vi "Scripting Save object.vi"(7 "Object type":T1=21751 items=[".NET Container"=2125, ".NET Refnum"=3441, "2D Picture"=3508, "3D Picture"=23776, "ActiveX Container"=2072, "Application Refnum"=3412, "Array (classic)"=3300, "Array (modern)"=21608, "Array Interface Control"=23777, "Atmospheric Tank (classic)"=3070, "Atmospheric Tank (modern)"=21751, "Automation Refnum"=3410, "Bin 1"=3073, "Bin 2"=21755, "Byte Stream File Refnum"=3408, "CAN Channel (classic)"=3340, "CAN Channel (modern)"=21817, "CAN Channel (system)"=21966, "CAN Interface (classic)"=3339, "CAN Interface (modern)"=21815, "CAN Interface (system)"=21964, "CAN Task (classic)"=3470, "CAN Task (modern)"=21789, "CAN Task (system)"=21963, "Cancel Button (modern)"=21739, "Cancel Button (system)"=3131, "Checkbox (classic)"=3117, "CheckBox (modern)"=21924, "Checkbox (system)"=3132, "Cluster (classic)"=3400, "Cluster (modern)"=21607, "Color Box"=3013, "Color Box Thin Border"=2905, "Color Ramp"=3022, "Combo Box (classic)"=3304, "Combo Box (modern)"=21604, "Combo Box (system)"=21917, "Control Refnum"=3419, "DAQmx Analog Trigger Source (classic)"=3336, "DAQmx Analog Trigger Source (modern)"=21774, "DAQmx Analog Trigger Source (system)"=21951, "DAQmx Device Name (classic)"=3318, "DAQmx Device Name (modern)"=21773, "DAQmx Device Name (system)"=21950, "DAQmx Global Channel (classic)"=3443, "DAQmx Global Channel (modern)"=21770, "DAQmx Global Channel (system)"=21957, "DAQmx Physical Channel (classic)"=3335, "DAQmx Physical Channel (modern)"=21777, "DAQmx Physical Channel (system)"=21954, "DAQmx Scale Name (classic)"=3317, "DAQmx Scale Name (modern)"=21775, "DAQmx Scale Name (system)"=21952, "DAQmx Switch (classic)"=3337, "DAQmx Switch (modern)"=21776, "DAQmx Switch (system)"=21953, "DAQmx Task Name (classic)"=3442, "DAQmx Task Name (modern)"=21778, "DAQmx Task Name (system)"=21959, "DAQmx Terminal (classic)"=3319, "DAQmx Terminal (modern)"=21781, "DAQmx Terminal (system)"=21955, "Data Log File Refnum"=3402, "DataSocket Refnum"=3417, "Device Refnum"=3405, "Dial (classic)"=3050, "Dial (modern)"=21732, "Digital Data (classic)"=3210, "Digital Data (modern)"=21216, "Digital Waveform Graph (classic)"=3511, "Digital Waveform Graph (modern)"=21718, "Dlg Horiz Scrollbar"=21905, "Dlg Numeric 1"=2100, "Dlg Numeric 2"=3006, "Dlg String"=2110, "Dlg Vert Scrollbar"=21906, "Down Arrow"=3824, "Down Bow Valve (flat)"=3707, "Down Bow Valve (outline)"=3807, "Down Bow Valve (shaded)"=21767, "Down Rect Valve (flat)"=3706, "Down Rect Valve (outline)"=3806, "Down Rect Valve (shaded)"=21766, "Down Tee (flat)"=3818, "Down Tee (shaded)"=3718, "Enum (classic)"=3023, "Enum (modern)"=21605, "Enum (system)"=3062, "Event Callback Refnum"=3435, "Exchanger"=3828, "FieldPoint IO Point (classic)"=3439, "FieldPoint IO Point (modern)"=21784, "FIFO Refnum"=3474, "File Path Control (classic)"=3203, "File Path Control (modern)"=21730, "File Path Control (system)"=21922, "File Path Indicator (classic)"=3204, "File Path Indicator (modern)"=21731, "Flat Box"=3602, "Flat Circle"=3605, "Flat Down Triangle"=3623, "Flat Frame"=3608, "Flat Left Triangle"=3620, "Flat Right Triangle"=3621, "Flat Round Button"=3102, "Flat Rounded Box"=3611, "Flat Sequence Structure"=2069, "Flat Square Button"=3103, "Flat Up Triangle"=3622, "Framed Color Box (classic)"=3008, "Framed Color Box (modern)"=21019, "Furnace"=3829, "Gauge (classic)"=3040, "Gauge (modern)"=21009, "Hopper 1"=21754, "Hopper 2"=3072, "Horiz Line"=3821, "Horiz Pipe (flat)"=3810, "Horiz Pipe (shaded)"=3710, "Horizontal Button Box"=3636, "Horizontal Fill Slide (classic)"=3012, "Horizontal Fill Slide (modern)"=21100, "Horizontal Graduated Bar"=21106, "Horizontal Pointer Slide (classic)"=3011, "Horizontal Pointer Slide (modern)"=21101, "Horizontal Pointer Slide (system)"=21902, "Horizontal Progress Bar (modern)"=21102, "Horizontal Progress Bar (system)"=21910, "Horizontal Scrollbar"=21110, "Horizontal Slide (classic)"=3010, "Horizontal Slide (system)"=21904, "Horizontal Slide Switch"=3114, "Horizontal Smooth Box"=3633, "Horizontal Splitter Bar (Classic)"=21863, "Horizontal Splitter Bar (System)"=21865, "Horizontal Switch"=3108, "Horizontal Tank"=3071, "Horizontal Toggle Switch (classic)"=3110, "Horizontal Toggle Switch (modern)"=21700, "IMAQ Session"=3415, "Intensity Chart (classic)"=3509, "Intensity Chart (modern)"=21719, "Intensity Graph (classic)"=3510, "Intensity Graph (modern)"=21720, "IrDA Network Connection Refnum"=3450, "IVI Logical Name (classic)"=3414, "IVI Logical Name (modern)"=21736, "Knob (classic)"=3005, "Knob (modern)"=21000, "Label (modern)"=21960, "Label (system)"=21961, "Labeled Oblong Button"=3125, "Labeled Rectangular Button"=3124, "Labeled Round Button"=3122, "Labeled Square Button"=3123, "LED Button"=3116, "Left Arrow"=3826, "Left Bow Valve (flat)"=3701, "Left Bow Valve (outline)"=3801, "Left Bow Valve (shaded)"=21761, "Left Down Elbow (flat)"=3811, "Left Down Elbow (shaded)"=3711, "Left Pump (flat)"=3813, "Left Pump (shaded)"=3713, "Left Rect Valve (flat)"=3700, "Left Rect Valve (outline)"=3800, "Left Rect Valve (shaded)"=21760, "Left Tee (flat)"=3809, "Left Tee (shaded)"=3709, "Left Up Elbow (flat)"=3808, "Left Up Elbow (shaded)"=3708, "Line (chiseled, system)"=3632, "Line (chiseled, thick)"=3630, "Line (chiseled, thin)"=3627, "Line (thick)"=3629, "Line (thin)"=3626, "Line with Arrow (thick)"=3631, "Line with Arrow (thin)"=3628, "Listbox (classic)"=21806, "Listbox (modern)"=21792, "Listbox (system)"=21805, "Lowered Box (thick)"=3635, "Lowered Rounded Box"=3638, "Menu Refnum"=3413, "Menu Ring (classic)"=3018, "Menu Ring (modern)"=21600, "Menu-Popup Ring"=3017, "Meter (classic)"=3030, "Meter (modern)"=21008, "Mixed Checkbox (system)"=21333, "Mixed Signal Graph"=21721, "Motion Resource (classic)"=3448, "Motion Resource (modern)"=21787, "Motor (flat)"=3820, "Motor (shaded)"=3720, "Multi-Segment Pipe"=23780, "Multicolumn Listbox (classic)"=21799, "Multicolumn Listbox (modern)"=21791, "Multicolumn Listbox (system)"=21798, "Notifier Refnum"=3423, "Numeric Control (classic)"=3000, "Numeric Control (modern)"=21003, "Numeric Control (system)"=21919, "Numeric Indicator (classic)"=3001, "Numeric Indicator (modern)"=21004, "Occurrence Refnum"=3406, "OK Button (modern)"=21738, "OK Button (system)"=3130, "Open Application Reference"=8012, "Open VI Object Reference"=8013, "Open VI Reference"=8010, "PassControl"=1968, "Pict Ring (classic)"=3015, "Pict Ring (modern)"=21602, "Pict Ring (system)"=21925, "PixMap"=3505, "PixMap (warning: dangerous)"=3507, "Platform Flat Square Button"=3134, "Plug-In Control"=21820, "Preserve Run-Time Class"=8018, "Pressure Tank (flat)"=3075, "Pressure Tank (shaded)"=21753, "Preview Queue Element"=9112, "Pulldown Menu Ring"=3061, "Push Button"=21001, "Queue Refnum"=3424, "Radio Button (system)"=3133, "Radio Buttons (classic)"=22003, "Radio Buttons (modern)"=22001, "Radio Buttons (system)"=22002, "Raised Box (classic)"=3600, "Raised Box (modern)"=3637, "Raised Circle"=3603, "Raised Down Triangle"=3615, "Raised Frame"=3606, "Raised Left Triangle"=3612, "Raised Right Triangle"=3613, "Raised Rounded Box"=3609, "Raised Up Triangle"=3614, "Recessed Box"=3601, "Recessed Circle"=3604, "Recessed Down Triangle"=3619, "Recessed Frame (modern)"=3607, "Recessed Frame (system)"=3624, "Recessed Left Triangle"=3616, "Recessed Menu Ring"=3019, "Recessed Right Triangle"=3617, "Recessed Rounded Box"=3610, "Recessed Up Triangle"=3618, "RecomposeUnlockDataValRef (warning: dangerous)"=2407, "Rectangular Stop Button"=3128, "Right Arrow"=3825, "Right Bow Valve (flat)"=3705, "Right Bow Valve (outline)"=3805, "Right Bow Valve (shaded)"=21765, "Right Down Elbow (flat)"=3817, "Right Down Elbow (shaded)"=3717, "Right Pump (flat)"=3819, "Right Pump (shaded)"=3719, "Right Rect Valve (flat)"=3704, "Right Rect Valve (outline)"=3804, "Right Rect Valve (shaded)"=21764, "Right Tee (flat)"=3815, "Right Tee (shaded)"=3715, "Right Up Elbow (flat)"=3814, "Right Up Elbow (shaded)"=3714, "Rocker"=21002, "Rotary Feeder"=3830, "Round Button"=3100, "Round LED (classic)"=3120, "Round LED (modern)"=21012, "Round Light"=3104, "Round Push Button"=3118, "Round Push Button (profile)"=3112, "Round Radio Button"=3106, "Round Stop Button"=3127, "Shared Variable Control (classic)"=3472, "Shared Variable Control (modern)"=21814, "Simple Horizontal Slide"=3003, "Simple Numeric"=2900, "Simple String"=2115, "Simple Vertical Slide"=3002, "Slide Switch"=21011, "Spin Control (system)"=21900, "Split Button"=21020, "Split Number"=1170, "Square Button"=3101, "Square LED (classic)"=3121, "Square LED (modern)"=21013, "Square Light"=3105, "Square Push Button"=3119, "Square Push Button (profile)"=3113, "Square Radio Button"=3107, "Static VI Reference"=2084, "Stop"=1350, "Stop Button"=21230, "Stop Stream"=23807, "String Control (classic)"=3200, "String Control (modern)"=21701, "String Control (system)"=21920, "String Indicator (classic)"=3201, "String Indicator (modern)"=21702, "SubPanel (Classic)"=21811, "SubPanel (System)"=21823, "Tab Control (classic)"=3330, "Tab Control (modern)"=3332, "Tab Control (system)"=3331, "Table (classic)"=21796, "Table (modern)"=21790, "Table (system)"=21797, "Tag Attribute Ring"=2063, "Tank (classic)"=3020, "Tank (modern)"=21006, "TCP Network Connection Refnum"=3407, "Text & Pict Ring (classic)"=3016, "Text & Pict Ring (modern)"=21603, "Text Button"=21015, "Text Ring (classic)"=3014, "Text Ring (modern)"=21601, "Text Ring (system)"=3060, "Thermometer (classic)"=3021, "Thermometer (modern)"=21007, "Time Stamp Control (classic)"=5555, "Time Stamp Control (modern)"=21913, "Time Stamp Control (system)"=21967, "Time Stamp Indicator (classic)"=5556, "Time Stamp Indicator (modern)"=21914, "Tree (classic)"=21819, "Tree (modern)"=21793, "Tree (system)"=21794, "UDP Network Connection Refnum"=3418, "Unleak Variant Value Reference"=2411, "Up Arrow"=3823, "Up Bow Valve (flat)"=3703, "Up Bow Valve (outline)"=3803, "Up Bow Valve (shaded)"=21763, "Up Rect Valve (flat)"=3702, "Up Rect Valve (outline)"=21762, "Up Rect Valve (shaded)"=3802, "Up Tee (flat)"=3812, "Up Tee (shaded)"=3712, "User Defined Refnum"=3428, "User Defined Refnum Tag (classic)"=3429, "User Defined Refnum Tag (modern)"=21745, "User Defined Refnum Tag Flatten (classic)"=3454, "User Defined Refnum Tag Flatten (modern)"=21747, "User Defined Tag (classic)"=3329, "User Defined Tag (modern)"=21749, "User Item"=3506, "Vert Line"=3822, "Vert Pipe (flat)"=3816, "Vert Pipe (shaded)"=3716, "Vert Rocker"=21740, "Vertical Fill Slide (classic)"=3009, "Vertical Fill Slide (modern)"=21014, "Vertical Graduated Bar"=21107, "Vertical Pointer Slide (classic)"=3007, "Vertical Pointer Slide (modern)"=21017, "Vertical Pointer Slide (system)"=21901, "Vertical Progress Bar (modern)"=21104, "Vertical Progress Bar (system)"=21909, "Vertical Scrollbar"=21111, "Vertical Slide"=3004, "Vertical Slide (system)"=21903, "Vertical Slide Switch (classic)"=3115, "Vertical Slide Switch (modern)"=21741, "Vertical Smooth Box"=3634, "Vertical Splitter Bar"=21860, "Vertical Splitter Bar (Classic)"=21862, "Vertical Splitter Bar (System)"=21864, "Vertical Switch"=3109, "Vertical Toggle Switch (classic)"=3111, "Vertical Toggle Switch (modern)"=21005, "VI Refnum"=3422, "VI Server Reference"=2091, "VISA resource name (classic)"=3409, "VISA resource name (modern)"=21737, "Waveform Chart (classic)"=3501, "Waveform Chart (modern)"=21717, "Waveform Graph (classic)"=3504, "Waveform Graph (modern)"=21703, "XY Graph (classic)"=3500, "XY Graph (modern)"=21716], 8 "error in":errorcluster, 11 "Temp Folder Path":path=path "C:/Users/fibergss/Desktop/Special Demos/Move Objects Demo/Objects/temp") -> (0 "error out":errorcluster={"status"=TRUE, "code"=1, "source"="Invoke Node in Scripting Save object.vi\n<APPEND>\nMethod Name: <b>Save:Instrument</b>"}, 3 "New VI Path Out":path=path "/Atmospheric Tank (modern).vi")   [LabVIEW 2012]
uses:
  Controls/Object Names.ctl
  <vilib>/Utility/miscctls.llb/LVPointTypeDef.ctl
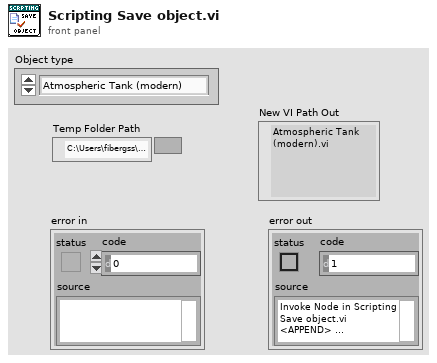
[diagram p1: front panel]
types:
  T1 = typedef "Object Names.ctl" = u16
  T2 = typedef "LVPointTypeDef.ctl" = cluster{"Horizontal":i16, "Vertical":i16}
  T3 = typedef "LVRectTypeDef.ctl" = cluster{"Left":i16, "Top":i16, "Right":i16, "Bottom":i16}
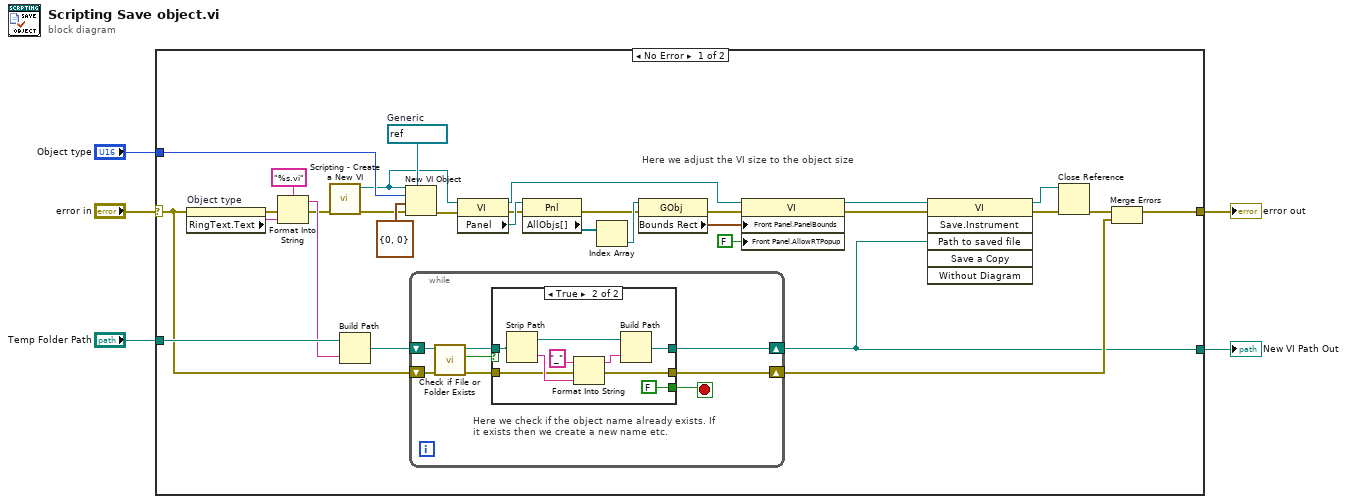
[diagram p0: block diagram]
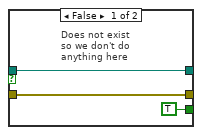
[diagram p2: hidden frame]
diagram:
  n1 = case shown="No Error" "error in" {
    selector: "error in" -> [w14 w57]
    tunnel: "Temp Folder Path" -> [w36 _]
    tunnel: [w9 _] -> w4
    tunnel: "Object type" -> [w35 _]
    tunnel: [w11 w57] -> w2
    frame No Error {
      w30 = refnum<vi> refnum  # Generic
      # "Here we adjust the VI size to the object size"
      n2 = property on="Object type" class="Ring (strict)"(error in=w14) -> (error out=w32:errorcluster, "RingText.Text"=w34:string)  [unwired: 1 in, 1 out]
      n3 = Format Into String(format string="%s.vi", error in=w32, w34) -> (resulting string=w33:string, error out=w31:errorcluster)  [unwired: 1 in]
      n4 = call "Scripting - Create a New VI.vi"("error in"=w31) -> ("error out"=w28:errorcluster, "VI Ref Out"=w25:refnum<vi>)  [unwired: 9 in]
      n5 = Build Path(base path=w36, name or relative path=w33) -> (appended path=w10:path)
      n6 = New VI Object(vi object class=w30, owner refnum=w25, style=w35, position/next to=T2 {"Horizontal"=0, "Vertical"=0} ("location"), 8:w28) -> (0:w16:errorcluster)  [unwired: 3 in, 1 out]
      n7 = while {
        shift-right: [w38] -> w9
        shift-left: w10 -> [w43]
        shift-right: [w39] -> w13
        shift-left: w14 -> [w44]
        stop <- w37 stop-if-true
        # "Here we check if the object name already exists. If it exists then we create a new name etc."
        n8 = call <vilib>:"Check if File or Folder Exists.vi"("error in (no error)"=w44, "path"=w43) -> ("error out"=w42:errorcluster, "file or folder exists?"=w41:bool, "dup path"=w40:path)  [unwired: 7 in]
        n9 = case shown="True" w41 {
          tunnel: w42 -> [w47 w52]
          tunnel: w40 -> [w45 w56]
          tunnel: [w47 w51] -> w39
          tunnel: [w45 w50] -> w38
          tunnel: [TRUE FALSE] -> w37
          frame False {
            # "Does not exist\nso we don't do\nanything here"
          }
          frame True {
            n10 = Strip Path(path=w56) -> (stripped path=w53:path, name=w55:string)
            n11 = Format Into String(initial string="_", error in=w52, w55) -> (resulting string=w54:string, error out=w51:errorcluster)  [unwired: 1 in]
            n12 = Build Path(base path=w53, name or relative path=w54) -> (appended path=w50:path)
          }
        }
      }
      n13 = property class="VI"(reference=w25, error in=w16) -> (reference out=w21:refnum<vi>, error out=w20:errorcluster, "Panel"=w24:refnum<vi>)
      n14 = property class="Pnl"(reference=w24, error in=w20) -> (error out=w19:errorcluster, "AllObjs[]"=w22:refnum<vi>[])  [unwired: 1 out]
      n15 = Index Array(array=w22) -> (element=w23:refnum<vi>)  [unwired: 1 in]
      n16 = property class="GObj"(reference=w23, error in=w19) -> (error out=w18:errorcluster, "Bounds Rect"=w17:T3)  [unwired: 1 out]
      n17 = property class="VI"(reference=w21, error in=w18, "Front Panel.PanelBounds"=w17, "Front Panel.AllowRTPopup"=FALSE ("Front Panel Window:Allow Runtime PopUp")) -> (reference out=w7:refnum<vi>, error out=w15:errorcluster)
      n18 = invoke class="VI" method="Save.Instrument"(reference=w7, error in=w15, "Path to saved file"=w9) -> (reference out=w27:refnum<vi>, error out=w26:errorcluster)  [unwired: 3 in, 4 out]
      n19 = Close Reference(reference=w27, error in (no error)=w26) -> (error out=w12:errorcluster)
      n20 = Merge Errors(w12, w13) -> (w11:errorcluster)
    }
    frame Error {
    }
  }
  "error out" <- w2
  "New VI Path Out" <- w4
